vi "Untitled 1 (SubVI).vi"(1 "Numeric 2":dbl, 2 "Enum":T1(ring), 3 "Numeric":dbl) -> (0 "Numeric 3":dbl)   [LabVIEW 2009]
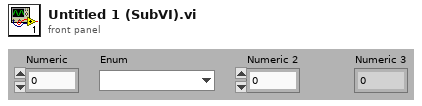
[diagram p1: front panel]
types:
  T1 = enum16{"", "ADD", "SUBTRACT", "DIVIDE", "MULTIPLY"}
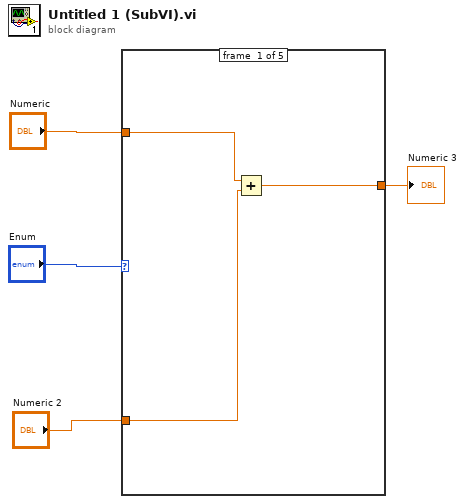
[diagram p0: block diagram]
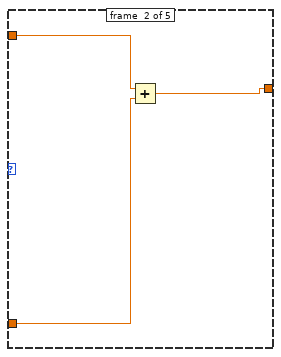
[diagram p2: hidden frame]
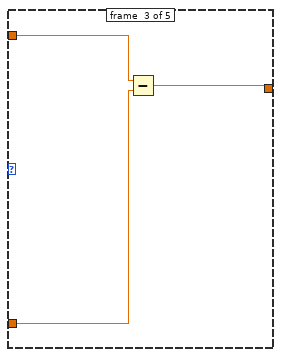
[diagram p3: hidden frame]
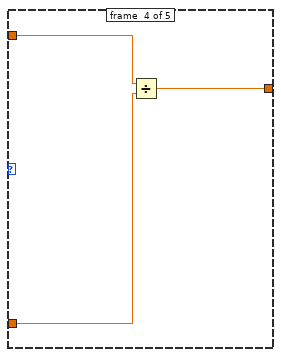
[diagram p4: hidden frame]
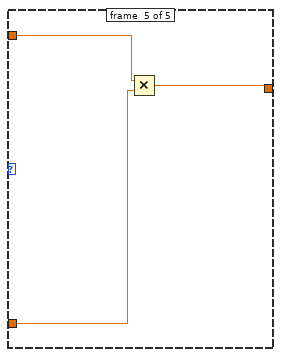
[diagram p5: hidden frame]
diagram:
  n1 = case shown="\"MULTIPLY\"" "Enum" {
    tunnel: "Numeric" -> [w7 w10 w13 w16 w19]
    tunnel: "Numeric 2" -> [w6 w9 w12 w15 w18]
    tunnel: [w5 w8 w11 w14 w17] -> w4
    frame #0 {
      n2 = Add(x=w7, y=w6) -> (x+y=w5:dbl)
    }
    frame #1 {
      n3 = Add(x=w10, y=w9) -> (x+y=w8:dbl)
    }
    frame #2 {
      n4 = Subtract(x=w13, y=w12) -> (x-y=w11:dbl)
    }
    frame #3 {
      n5 = Divide(x=w16, y=w15) -> (x/y=w14:dbl)
    }
    frame #4 {
      n6 = Multiply(x=w19, y=w18) -> (x*y=w17:dbl)
    }
  }
  "Numeric 3" <- w4
